vi "ProgressControlOvershootTest.vi"(2 "Array IN":dbl[](array[numeric]), 9 "Sample":dbl) -> (16 "Stable":bool)   [LabVIEW 2009]
panel:
  # "INPUT"
  # "OUTPUT"
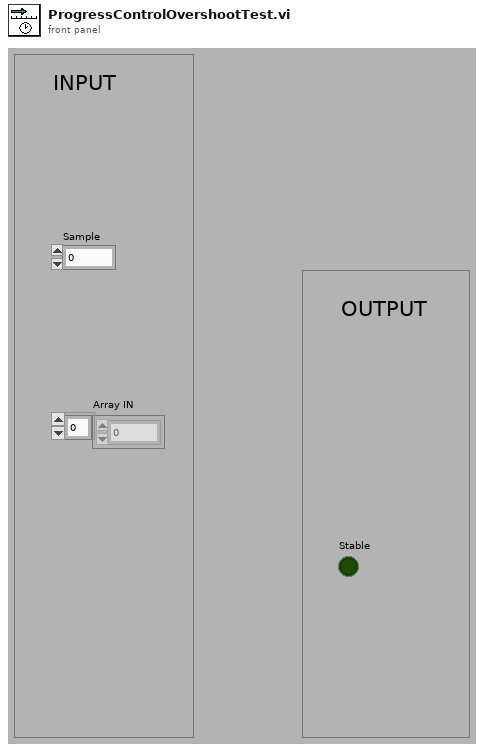
[diagram p1: front panel]
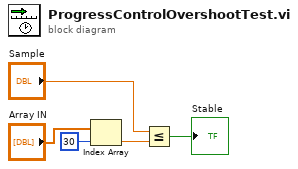
[diagram p0: block diagram]
diagram:
  n1 = Index Array(array="Array IN", index=30) -> (element=w4:dbl)
  n2 = Less Or Equal?(x="Sample", y=w4) -> (x <= y?=→"Stable":bool)
